vi "ReportPart1.vi"(6 "试验项目":enum32{"右工位"}(ring), 8 "error in":errorcluster, 9 "索引IN":i32, 10 "合格":T1, 11 "report in":refnum<class "NI_report.lvclass">) -> (0 "error out 2":errorcluster caption="error out", 2 "索引OUT":i32, 3 "report out":refnum<class "NI_report.lvclass">)   [LabVIEW 2020]
uses:
  <vilib>/Utility/NIReport.llb/NI_report.lvclass
  OK1.ctl
  <vilib>/Utility/NIReport.llb/image depth.ctl
  <vilib>/addons/_office/_exclsub.llb/font.ctl
  Global_Variable/A131258.vi
  <vilib>/Utility/NIReport.llb/Append Report Text (str wrap).vi
  Global_Variable/Global.vi
  <vilib>/addons/_office/word.llb/Word Easy Table (str).vi
  <vilib>/Utility/NIReport.llb/NI_ReportGenerationCore.lvlib
  <vilib>/addons/_office/NI_ReportGenerationToolkit.lvlib
  <vilib>/Utility/NIReport.llb/Word/NI_Word.lvclass
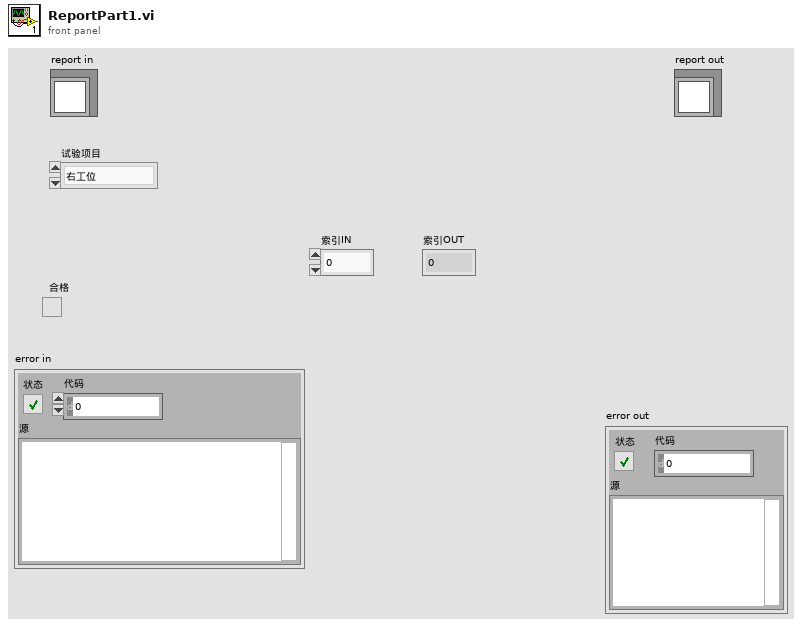
[diagram p1: front panel]
types:
  T1 = typedef "OK1.ctl" = bool
  T2 = cluster{"Charset (-1)":i16, "Weight (-1)":i16, "Name":string, "Size":string}
  T3 = cluster{"Italic":enum16{"Italic Unchanged", "Italic On", "Italic Off"}, "Strike Through":enum16{"Strike Through Unchanged", "Strike Through On", "Strike Through Off"}, "Underline":enum16{"Underline Unchanged", "Underline On", "Underline Off"}, "Bold":enum16{"Bold Unchanged", "Bold On", "Bold Off"}}
  T4 = typedef "NI_ReportGenerationToolkit.lvlib/font.ctl" = cluster{"font name":string, "font size":dbl, "bold":u16, "italic":u16, "underline":u16, "strike through":u16, "font color":u32}
  T5 = typedef "NI_ReportGenerationCore.lvlib/image depth.ctl" = u16
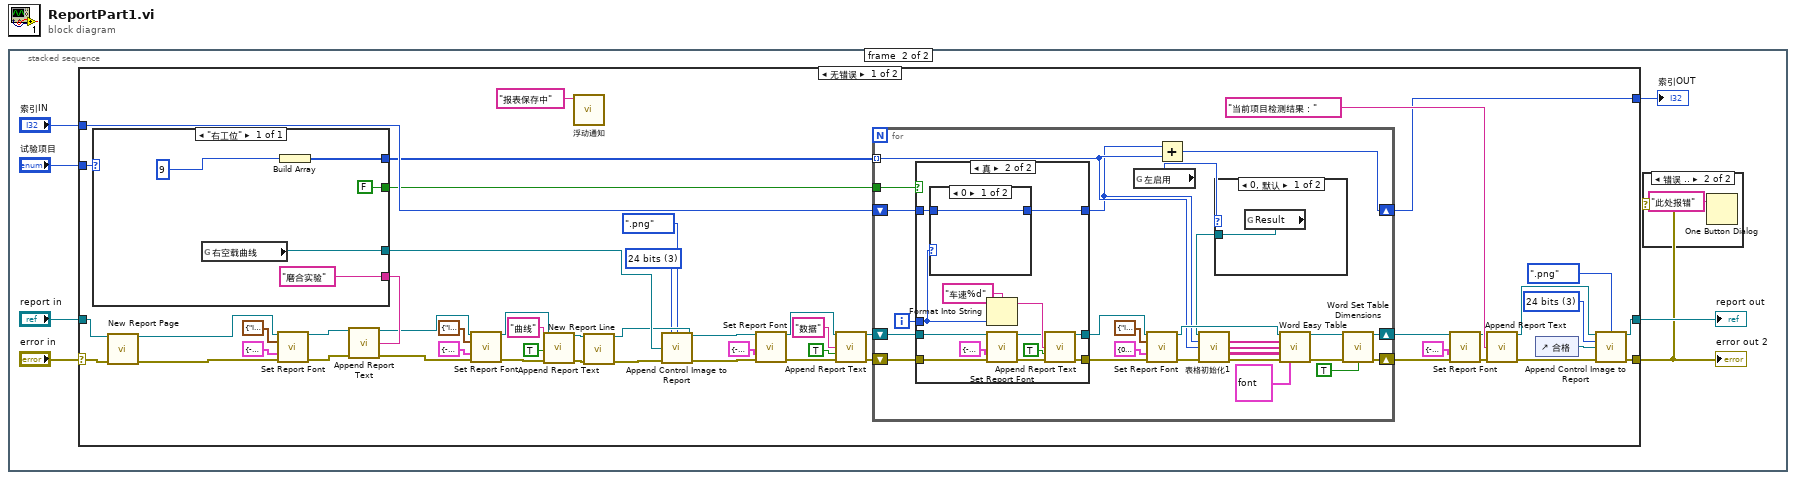
[diagram p0: block diagram]
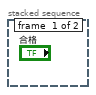
[diagram p2: hidden frame]
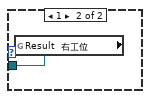
[diagram p4: hidden frame]
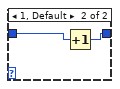
[diagram p6: hidden frame]
diagram:
  n1 = stacked-sequence {
    frame #0 {
    }
    frame #1 {
      n2 = case shown="无错误" "error in" {
        selector: "error in" -> [w53 w115]
        tunnel: [w48 w115] -> w1
        tunnel: "索引IN" -> [w20 w114]
        tunnel: "试验项目" -> [w23 _]
        tunnel: [w17 w114] -> w4
        tunnel: [w22 w113] -> w3
        tunnel: "report in" -> [w21 w113]
        frame No Error {
          w36 = T5 3 items=["B&W", "4 bits", "8 bits", "24 bits"] ("image depth")
          w46 = T5 3 items=["B&W", "4 bits", "8 bits", "24 bits"] ("image depth")
          n3 = case shown="\"右工位\"" w23 {
            tunnel: [w109] -> w39
            tunnel: ["磨合实验" ("text")] -> w57
            tunnel: [w111] -> w19
            tunnel: [FALSE] -> w16
            frame "右工位" {
              n4 = global read "A131258.vi" "右空载曲线"() -> (w109:refnum<vi>)
              n5 = Build Array(9) -> (w111:i32[])
            }
          }
          n6 = call-dynamic "New Report Page.vi"("report in"=w21, "error in (no error)"=w53) -> ("report out"=w51:refnum<class "NI_report.lvclass">, "error out"=w52:errorcluster)  [unwired: 12 in]
          n7 = call-dynamic "Set Report Font.vi"("report in"=w51, "text options"=T3 {"Italic"=enum."Italic Unchanged", "Strike Through"=enum."Strike Through Unchanged", "Underline"=enum."Underline Unchanged", "Bold"=enum."Bold On"}, "font settings"=T2 {"Charset (-1)"=-1, "Weight (-1)"=-1, "Name"="楷体", "Size"="16 "}, "error in (no error)"=w52) -> ("report out"=w60:refnum<class "NI_report.lvclass">, "error out"=w59:errorcluster)  [unwired: 9 in, 1 out]
          n8 = call-poly <vilib>:"Append Report Text.vi"("report in"=w60, "text"=w57, "error in (no error)"=w59) -> ("report out"=w55:refnum<class "NI_report.lvclass">, "error out"=w54:errorcluster)  [unwired: 9 in, 2 out]
          n9 = call-dynamic "Set Report Font.vi"("report in"=w55, "text options"=T3 {"Italic"=enum."Italic Unchanged", "Strike Through"=enum."Strike Through Unchanged", "Underline"=enum."Underline Unchanged", "Bold"=enum."Bold Off"}, "font settings"=T2 {"Charset (-1)"=-1, "Weight (-1)"=-1, "Name"="宋体", "Size"="12"}, "error in (no error)"=w54) -> ("report out"=w30:refnum<class "NI_report.lvclass">, "error out"=w27:errorcluster)  [unwired: 9 in, 1 out]
          n10 = call-poly <vilib>:"Append Report Text.vi"("report in"=w30, "text"="曲线", "append on new line? (F)"=TRUE, "error in (no error)"=w27) -> ("report out"=w29:refnum<class "NI_report.lvclass">, "error out"=w28:errorcluster)  [unwired: 8 in, 2 out]
          n11 = call "浮动通知.vi"("通知内容"="报表保存中") -> ()  [unwired: 11 in]
          n12 = call-dynamic "New Report Line.vi"("report in"=w29, "error in (no error)"=w28) -> ("report out"=w37:refnum<class "NI_report.lvclass">, "error out"=w38:errorcluster)  [unwired: 12 in]
          n13 = call-dynamic "Append Control Image to Report.vi"("report in"=w37, "image file type (.jpg)"=enum16{".jpg", ".png"}.".png", "image depth"=w36, "ctrl reference"=w39, "error in (no error)"=w38) -> ("report out"=w34:refnum<class "NI_report.lvclass">, "error out"=w33:errorcluster)  [unwired: 7 in, 2 out]
          n14 = call-dynamic "Set Report Font.vi"("report in"=w34, "font settings"=T2 {"Charset (-1)"=-1, "Weight (-1)"=-1, "Name"="微软雅黑", "Size"="12 "}, "error in (no error)"=w33) -> ("report out"=w15:refnum<class "NI_report.lvclass">, "error out"=w12:errorcluster)  [unwired: 10 in, 1 out]
          n15 = call-poly <vilib>:"Append Report Text.vi"("report in"=w15, "text"="数据", "append on new line? (F)"=TRUE, "error in (no error)"=w12) -> ("report out"=w11:refnum<class "NI_report.lvclass">, "error out"=w10:errorcluster)  [unwired: 8 in, 2 out]
          n16 = for {
            tunnel: w19 -> [w71] mode=indexing
            shift-right: [w86] -> w41
            shift-left: w11 -> [w69]
            shift-right: [w85] -> w40
            shift-left: w10 -> [w68]
            shift-right: [w70] -> w17
            shift-left: w20 -> [w63]
            tunnel: w16 -> [w64]
            i -> [w65]
            n17 = case shown="真" w64 {
              tunnel: w69 -> [w91 w98]
              tunnel: w68 -> [w90 w97]
              tunnel: [w91 w96] -> w67
              tunnel: [w90 w95] -> w66
              tunnel: w65 -> [_ w92]
              tunnel: w63 -> [w89 w94]
              tunnel: [w89 w93] -> w62
              frame False {
              }
              frame True {
                n18 = case shown="0" w92 {
                  tunnel: [w105 w106] -> w93
                  tunnel: w94 -> [w105 w107]
                  frame 0 {
                  }
                  frame 1, Default {
                    n19 = Increment(x=w107) -> (x+1=w106:i32)
                  }
                }
                n20 = Format Into String(format string="车速%d" ("格式字符串"), w92) -> (resulting string=w104:string)  [unwired: 2 in, 1 out]
                n21 = call-dynamic "Set Report Font.vi"("report in"=w98, "font settings"=T2 {"Charset (-1)"=-1, "Weight (-1)"=-1, "Name"="宋体", "Size"="12 "}, "error in (no error)"=w97) -> ("report out"=w103:refnum<class "NI_report.lvclass">, "error out"=w102:errorcluster)  [unwired: 10 in, 1 out]
                n22 = call-poly <vilib>:"Append Report Text.vi"("report in"=w103, "text"=w104, "append on new line? (F)"=TRUE, "error in (no error)"=w102) -> ("report out"=w96:refnum<class "NI_report.lvclass">, "error out"=w95:errorcluster)  [unwired: 8 in, 2 out]
              }
            }
            n23 = global read "Global.vi" "左启用"() -> (w61:i16)
            n24 = call-dynamic "Set Report Font.vi"("report in"=w67, "text options"=T3 {"Italic"=enum."Italic Unchanged", "Strike Through"=enum."Strike Through Unchanged", "Underline"=enum."Underline Unchanged", "Bold"=enum."Bold Unchanged"}, "font settings"=T2 {"Charset (-1)"=0, "Weight (-1)"=-1, "Name"="微软雅黑", "Size"="12 "}, "error in (no error)"=w66) -> ("report out"=w74:refnum<class "NI_report.lvclass">, "error out"=w73:errorcluster)  [unwired: 9 in, 1 out]
            n25 = Add(x=w62, y=w71) -> (x+y=w70:i32)
            n26 = case shown="0, 默认" w61 {
              tunnel: [w87 w88] -> w72
              frame 0, Default {
                n27 = global read "Global.vi" "Result"() -> (w87:refnum<vi>)
              }
              frame 1 {
                n28 = global read "Global.vi" "Result  右工位"() -> (w88:refnum<vi>)
              }
            }
            n29 = call "表格初始化1.vi"("表格引用"=w72, "索引"=w62, "长度"=w71, "错误输入（无错误）"=w73) -> ("行首字符串[]"=w76:string[], "列首字符串[]"=w75:string[], "文本数据"=w78:string[][], "错误输出"=w81:errorcluster)  [unwired: 7 in, 1 out]
            n30 = call-poly <vilib>:"Word Easy Table.vi"("report in"=w74, "row headers"=w76, "column headers"=w75, "data"=w78, "error in (no error)"=w81, "font"=T4 {"font name"="宋体", "font size"=12.0, "bold"=2, "italic"=2, "underline"=2, "strike through"=2, "font color"=16777216}) -> ("report out"=w79:refnum<class "NI_report.lvclass">, "error out"=w80:errorcluster)  [unwired: 7 in, 1 out]
            n31 = call <vilib>:"Word Set Table Dimensions.vi"("report in"=w79, "error in (no error)"=w80, "fit to page width? (F)"=TRUE) -> ("report out"=w86:refnum<class "NI_report.lvclass">, "error out"=w85:errorcluster)  [unwired: 11 in]
          }
          n32 = call-dynamic "Set Report Font.vi"("report in"=w41, "font settings"=T2 {"Charset (-1)"=-1, "Weight (-1)"=-1, "Name"="宋体", "Size"="16 "}, "error in (no error)"=w40) -> ("report out"=w44:refnum<class "NI_report.lvclass">, "error out"=w45:errorcluster)  [unwired: 10 in, 1 out]
          n33 = call-poly <vilib>:"Append Report Text.vi"("report in"=w44, "text"="当前项目检测结果：", "error in (no error)"=w45) -> ("report out"=w50:refnum<class "NI_report.lvclass">, "error out"=w49:errorcluster)  [unwired: 9 in, 2 out]
          n34 = control-ref of="合格"() -> (w18:refnum<vi>)
          n35 = call-dynamic "Append Control Image to Report.vi"("report in"=w50, "image file type (.jpg)"=enum16{".jpg", ".png"}.".png", "image depth"=w46, "ctrl reference"=w18, "error in (no error)"=w49) -> ("report out"=w22:refnum<class "NI_report.lvclass">, "error out"=w48:errorcluster)  [unwired: 7 in, 2 out]
        }
        frame Error {
        }
      }
      "error out 2" <- w1
      "索引OUT" <- w4
      "report out" <- w3
      n36 = case shown="错误 .." w1 {
        frame No Error {
        }
        frame Error {
          n37 = One Button Dialog(message="此处报错" ("消息")) -> ()  [unwired: 1 in, 1 out]
        }
      }
    }
  }
